vi "2-9.vi"() -> ()   [LabVIEW 2022 SP3]
panel:
  in  "簇":cluster{"布尔":bool, "数值":dbl, "数组":dbl[]}
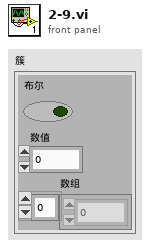
[diagram p1: front panel]
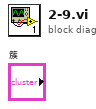
[diagram p0: block diagram]
diagram:
